vi "Demo Rearrange TDMS.vi"() -> ()   [LabVIEW 2015]
doc: "This VI will demonstrate the functionality fo the Rearrange TDMS Data. Follow the instructions on the front panel to use the VI.\n\n-----\nBrian Hoover (Hooovahh)"
uses:
  TDMS Functions/TDMS Group Information.ctl
panel:
  in  "New TDMS Path":path
  in  "TDMS File Path":path
  in  "Save As":bool
  in  "Cancel":bool
  in  "Channels in Group":i32(listbox)
  in  "Groups":string(combo)
  # "1) Run this VI.\n2) Provide a path to a TDMS file.\n3) Select a Group in the file.\n4) Drag and drop the Channels in the Group to make a new order for the channels.\n5) Provide a New TDMS path to save the reordered file to.\n6) Click Save As..."
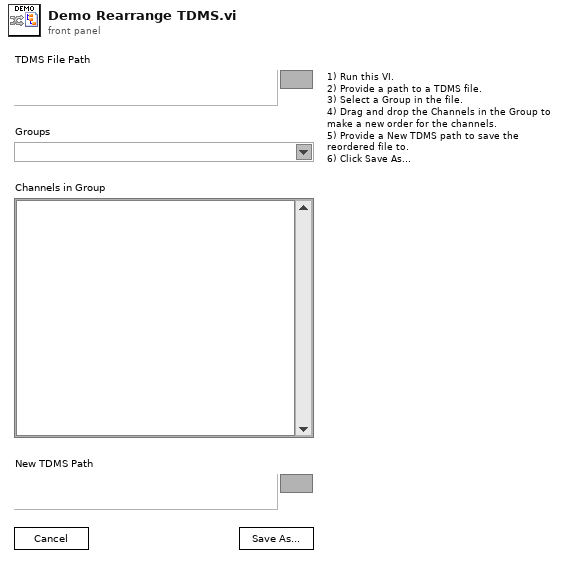
[diagram p1: front panel]
types:
  T1 = typedef "TDMS Group Information.ctl" = cluster{"Group Name":string, "Channel Names":string[]}
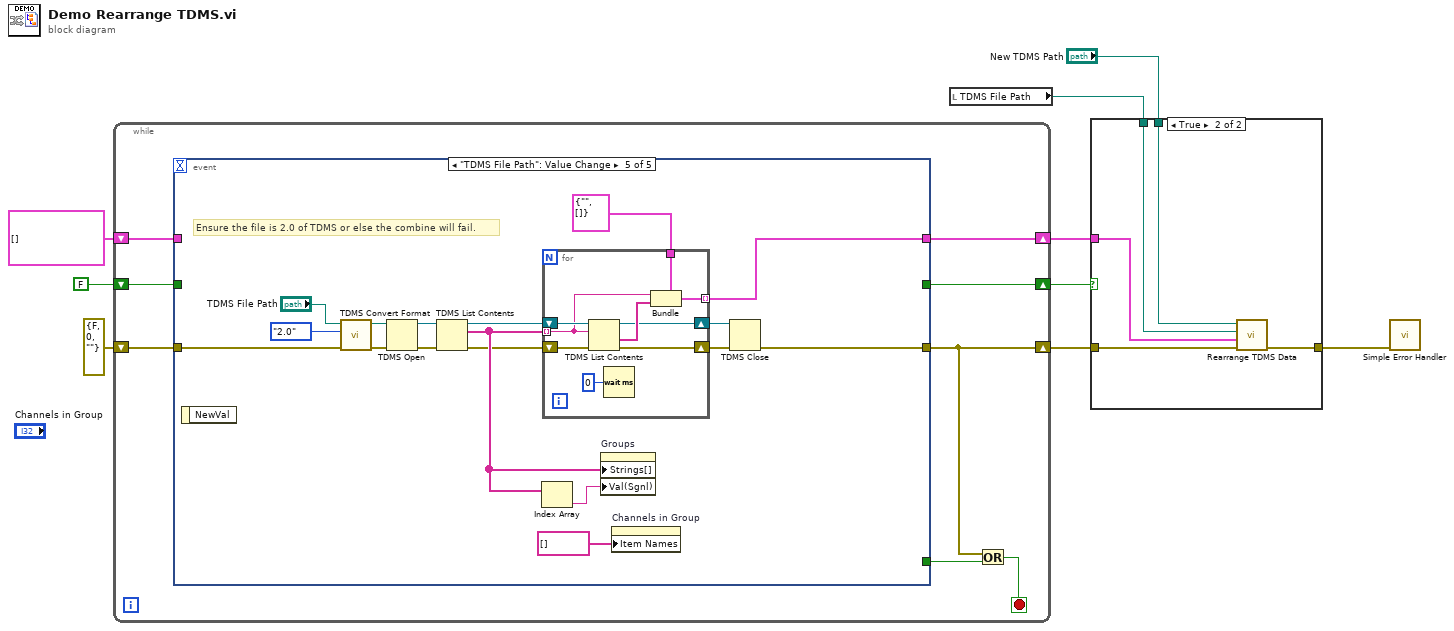
[diagram p0: block diagram]
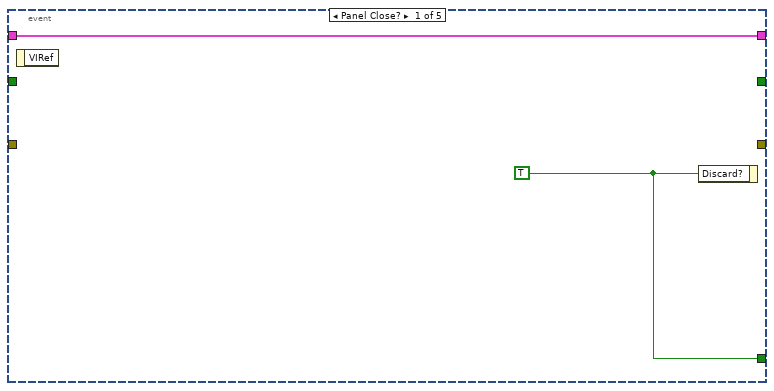
[diagram p3: hidden frame]
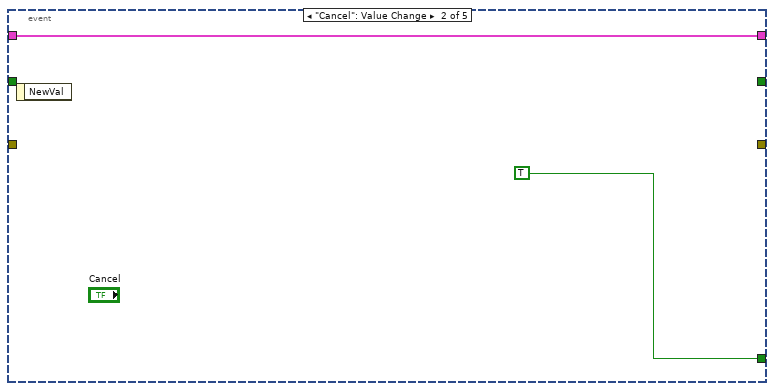
[diagram p4: hidden frame]
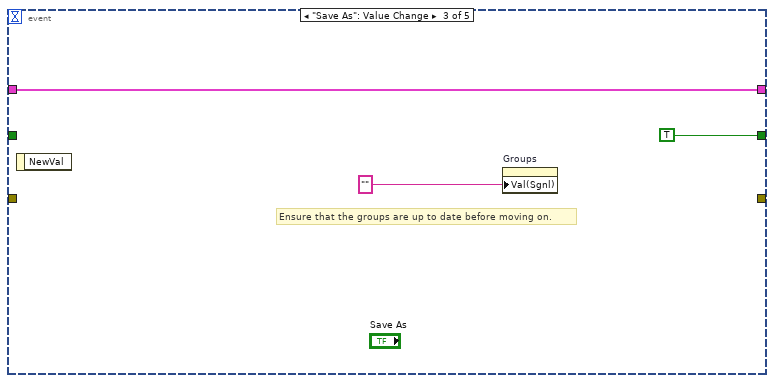
[diagram p5: hidden frame]
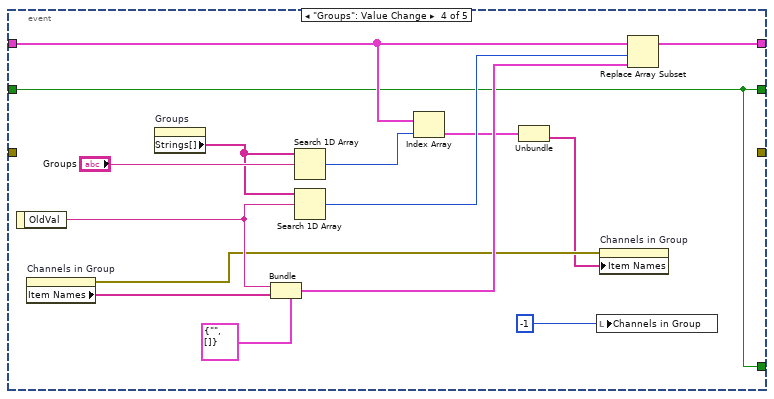
[diagram p6: hidden frame]
diagram:
  n1 = while {
    shift-right: [w15] -> w7
    shift-left: T1[] [] -> [w16]
    shift-right: [w14] -> w8
    shift-left: FALSE -> [w13]
    shift-right: [w10] -> w3
    shift-left: errorcluster {"status"=FALSE, "code"=0, "source"=""} ("error out") -> [w12]
    stop <- w11 stop-if-true
    n2 = event shown="[4] \"TDMS File Path\": Value Change" {
      selector: _ -> [_ _ _ _ _]
      dyn-events: _ -> [_ _ _ _ _]
      timeout: _ -> [_ _ _ _ _]
      tunnel: [w19 TRUE _ w27 _] -> w17
      tunnel: w16 -> [w18 w20 w24 w32 _]
      tunnel: [w18 w20 w24 w38 w44] -> w15
      tunnel: [_ _ TRUE w27 _] -> w14
      tunnel: w13 -> [_ _ _ w27 _]
      tunnel: [_ _ _ _ w43] -> w10
      tunnel: w12 -> [_ _ _ _ w42]
      event Panel Close? {
        w19 = TRUE
        n3 = event-data() -> ()  [unwired: 1 in, 1 out]
        n4 = event-data("Discard?"=w19) -> ()  [unwired: 1 in, 1 out]
      }
      event "Cancel": Value Change {
        n5 = event-data() -> ()  [unwired: 1 in, 1 out]
      }
      event "Save As": Value Change {
        # "Ensure that the groups are up to date before moving on."
        n6 = event-data() -> ()  [unwired: 1 in, 1 out]
        n7 = property on="Groups" class="CmbBox"("Val(Sgnl)"="") -> ()  [unwired: 2 in, 2 out]
      }
      event "Groups": Value Change {
        n8 = event-data() -> ("OldVal"=w34:string)  [unwired: 1 in]
        n9 = property on="Channels in Group" class="LstBox (strict)"() -> (error out=w29:errorcluster, "Item Names"=w37:string[])  [unwired: 2 in, 1 out]
        n10 = property on="Groups" class="CmbBox"() -> ("Strings[]"=w25:string[])  [unwired: 2 in, 2 out]
        n11 = Bundle(cluster=T1 {"Group Name"="", "Channel Names"=[]}, "Group Name"=w34, "Channel Names"=w37) -> (w35:T1)
        n12 = Search 1D Array(1D array=w25, element="Groups") -> (index of element=w31:i32)  [unwired: 1 in]
        n13 = Search 1D Array(1D array=w25, element=w34) -> (index of element=w36:i32)  [unwired: 1 in]
        n14 = Index Array(array=w32, index=w31) -> (element=w30:T1)
        n15 = Unbundle(w30) -> ("Channel Names"=w28:string[])  [unwired: 1 out]
        n16 = local write "Channels in Group"(-1 ("Channels in Group")) -> ()
        n17 = property on="Channels in Group" class="LstBox (strict)"(error in=w29, "Item Names"=w28) -> ()  [unwired: 1 in, 2 out]
        n18 = Replace Array Subset(array=w32, new element=w35, index=w36) -> (w38:T1[])
      }
      event "TDMS File Path": Value Change {
        # "Ensure the file is 2.0 of TDMS or else the combine will fail."
        n19 = event-data() -> ()  [unwired: 1 in, 1 out]
        n20 = call <vilib>:"TDMS Convert Format.vi"("error in (no error)"=w42, "target version"=enum16{"1.0", "2.0"}."2.0", "file path"="TDMS File Path") -> ("error out"=w53:errorcluster, "file path out"=w54:path)  [unwired: 3 in]
        n21 = TDMS Open(8:w53, 11:w54) -> (0:w45:errorcluster, 3:w46:refnum<k34>)  [unwired: 5 in]
        n22 = TDMS List Contents(4:w45, 7:w46) -> (0:w40:errorcluster, 2:w55:string[], 3:w47:refnum<k34>)  [unwired: 1 in, 1 out]
        n23 = Index Array(array=w55) -> (element=w56:string)  [unwired: 1 in]
        n24 = for {
          tunnel: w55 -> [w62] mode=indexing
          tunnel: T1 {"Group Name"="", "Channel Names"=[]} -> [w63]
          shift-right: [w60] -> w48
          shift-left: w47 -> [w64]
          shift-right: [w57] -> w49
          shift-left: w40 -> [w65]
          tunnel: [w58] -> w44 mode=indexing
          n25 = TDMS List Contents(4:w65, 6:w62, 7:w64) -> (0:w57:errorcluster, 1:w61:string[], 3:w60:refnum<k34>)  [unwired: 1 out]
          n26 = Wait (ms)(milliseconds to wait=u32 0) -> ()  [unwired: 1 out]
          n27 = Bundle(cluster=w63, "Group Name"=w62, "Channel Names"=w61) -> (w58:T1)
        }
        n28 = property on="Groups" class="CmbBox"("Strings[]"=w55, "Val(Sgnl)"=w56) -> ()  [unwired: 2 in, 2 out]
        n29 = property on="Channels in Group" class="LstBox (strict)"("Item Names"=string[] []) -> ()  [unwired: 2 in, 2 out]
        n30 = TDMS Close(8:w49, 11:w48) -> (0:w43:errorcluster)  [unwired: 1 out]
      }
    }
    n31 = Or(x=w10, y=w17) -> (x .or. y?=w11:bool)
  }
  n32 = local read "TDMS File Path"() -> (w1:path)
  n33 = case shown="True" w8 {
    tunnel: w7 -> [_ w67]
    tunnel: w1 -> [_ w71]
    tunnel: "New TDMS Path" -> [_ w70]
    tunnel: w3 -> [w66 w69]
    tunnel: [w66 w68] -> w2
    frame False {
    }
    frame True {
      n34 = call "Rearrange TDMS Data.vi"("error in (no error)"=w69, "TDMS Group Channel Order"=w67, "Existing TDMS Path"=w71, "New TDMS Path"=w70) -> ("error out"=w68:errorcluster)  [unwired: 7 in]
    }
  }
  n35 = call <vilib>:"Simple Error Handler.vi"("error in (no error)"=w2) -> ()  [unwired: 4 in, 5 out]
